vi "Glass Display Type Change.vi"(0 "Data To Glass Type":T1(ring)) -> ()   [LabVIEW 2013]
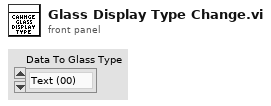
[diagram p1: front panel]
types:
  T1 = enum16{"Text (00)", "Shoot Status (01)", "Shoot Dist. (02)", "Pressure (03)", "Feed Dist. (04)", "Shutdown (99)"}
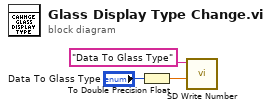
[diagram p0: block diagram]
diagram:
  n1 = To Double Precision Float(number="Data To Glass Type") -> (double precision float=w2:dbl)
  n2 = call <vilib>:"SD Write Number.vi"("Numeric"=w2, "Name"="Data To Glass Type") -> ()  [unwired: 8 in, 2 out]
